vi "Update Channels.vi"(6 "Settings":T1={"Step Values"=[], "Only Execute When Test Running"=TRUE, "Reset Sequence When Test Starts"=TRUE, "Current Sequence ID"=0, "Total Iterations"=0, "Current Step Start Timestamp"=0.0, "Number of Sequence Steps"=0, "Num of Analog Channels"=0, "Num of Digital Channels"=0, "Delay Before Starting Sequence"=0.0, "Show UI"=FALSE, "Time Remaining"=0.0, "Test Running"=FALSE, "Pause Timestamp"=0.0, "Default Analog Values"=[], "Default Digital Values"=[]}, 8 "error in":errorcluster, 9 "Analog":bool, 10 "Previous Number of Channels":i32=8, 11 "Plugin in":refnum<class "Sequencer with Output Values.lvclass">) -> (0 "error out":errorcluster, 1 "Channels to Remove":string[](array[string]), 2 "Updated Number of Channels":i32, 3 "Plugin out":refnum<class "Sequencer with Output Values.lvclass">, 5 "Channels to Add":refnum<class "Producer Channel.lvclass">[](array[class]))   [LabVIEW 2020, in "Sequencer with Output Values.lvlib" / "Sequencer with Output Values.lvclass"]
uses:
  Sequencer with Output Values.lvclass
  Params.ctl
  Step Settings.ctl
  <vilib>/FlexLogger/SDK/PluginSDK.lvlibp/PEFClasses/SDK/Producer Channel/Producer Channel.lvclass
  <vilib>/FlexLogger/SDK/PluginSDK.lvlibp/PEFClasses/SDK/Channel/Data Type.ctl
  Global Strings.vi
  <vilib>/FlexLogger/SDK/PluginSDK.lvlibp/PEFClasses/SDK/Producer Channel/Create Producer Channel.vi
  <vilib>/FlexLogger/SDK/PluginSDK.lvlibp/PEFClasses/SDK/Plugin/Plugin.lvclass
  <vilib>/FlexLogger/SDK/PluginSDK.lvlibp
  <vilib>/FlexLogger/SDK/PluginSDK.lvlibp/PEFClasses/SDK/Channel/Channel.lvclass
  C:/Program Files/National Instruments/LabVIEW 2024/vi.lib/FlexLogger/SDK/PluginSDK.lvlibp/PEFClasses/SDK/Plugin/Plugin.lvclass
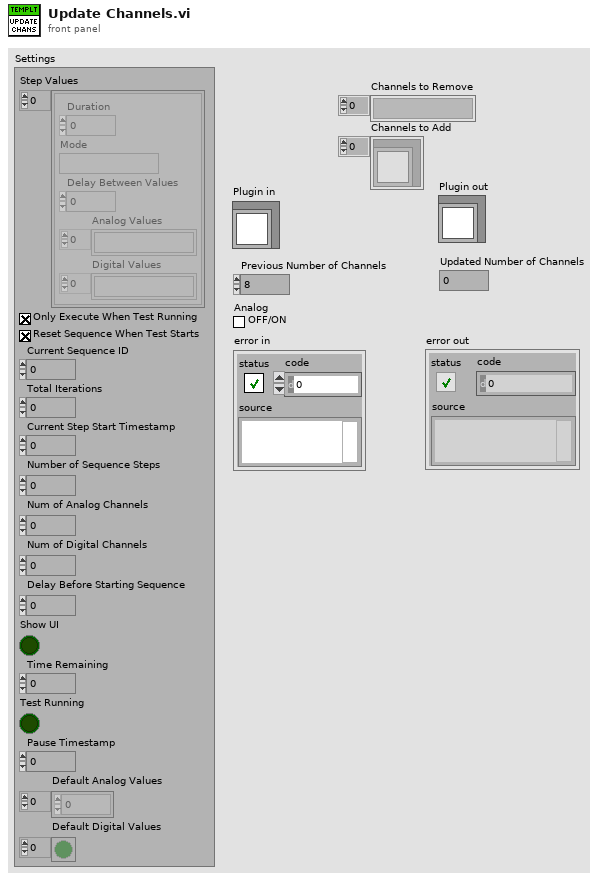
[diagram p1: front panel]
types:
  T1 = typedef "Sequencer with Output Values.lvlib/Sequencer with Output Values.lvclass/Params.ctl" = cluster{"Step Values":T2[], "Only Execute When Test Running":bool, "Reset Sequence When Test Starts":bool, "Current Sequence ID":u32, "Total Iterations":u32, "Current Step Start Timestamp":dbl, "Number of Sequence Steps":i32, "Num of Analog Channels":i32, "Num of Digital Channels":i32, "Delay Before Starting Sequence":dbl, "Show UI":bool, "Time Remaining":dbl, "Test Running":bool, "Pause Timestamp":dbl, "Default Analog Values":dbl[], "Default Digital Values":bool[]}
  T2 = typedef "Sequencer with Output Values.lvlib/Sequencer with Output Values.lvclass/Step Settings.ctl" = cluster{"Duration":dbl, "Mode":string, "Delay Between Values":dbl, "Analog Values":string[], "Digital Values":string[]}
  T3 = typedef "PluginSDK.lvlibp/Channel.lvclass/Data Type.ctl" = enum16{"Wfm (DBL)", "Wfm (Digital)"}
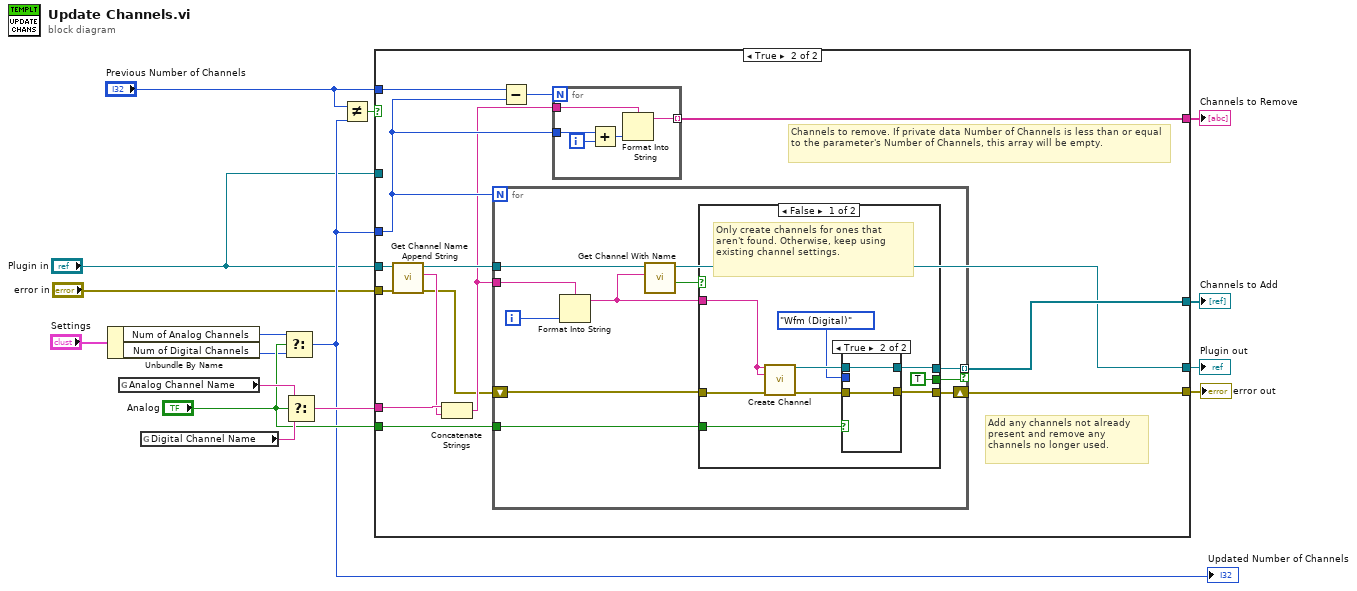
[diagram p0: block diagram]
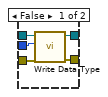
[diagram p3: hidden frame]
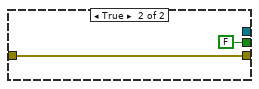
[diagram p4: hidden frame]
diagram:
  n1 = Unbundle By Name("Settings") -> ("Num of Analog Channels"=w4:i32, "Num of Digital Channels"=w3:i32)
  n2 = global read "Global Strings.vi" "Analog Channel Name"() -> (w14:string)
  n3 = global read "Global Strings.vi" "Digital Channel Name"() -> (w13:string)
  n4 = Select(t=w4, s="Analog", f=w3) -> (s? t:f=w8:i32)
  "Updated Number of Channels" <- w8
  n5 = Select(t=w14, s="Analog", f=w13) -> (s? t:f=w12:string)
  n6 = Not Equal?(x="Previous Number of Channels", y=w8) -> (x != y?=w16:bool)
  n7 = case shown="True" w16 {
    tunnel: "Previous Number of Channels" -> [_ w32]
    tunnel: w8 -> [_ w29]
    tunnel: "Plugin in" -> [w18 w25]
    tunnel: "error in" -> [w17 w21]
    tunnel: "Plugin in" -> [_ _]
    tunnel: [w18 w24] -> w11
    tunnel: [w17 w27] -> w10
    tunnel: w12 -> [_ w23]
    tunnel: "Analog" -> [_ w30]
    tunnel: [_ w28] -> w2
    tunnel: [_ w26] -> w1
    frame False {
    }
    frame True {
      # "Add any channels not already present and remove any channels no longer used."
      # "Channels to remove. If private data Number of Channels is less than or equal to the parameter's Number of Channels, this array will be empty."
      n8 = call "Get Channel Name Append String.vi"("error in (no error)"=w21, "Plugin In"=w25) -> ("error out"=w19:errorcluster, "Channel Append String"=w20:string, "Plugin Out"=w24:refnum<class "Sequencer with Output Values.lvclass">)  [unwired: 7 in]
      n9 = Concatenate Strings(w23, w20) -> (w22:string)
      n10 = for {
        N: w29 -> [_]
        tunnel: w24 -> [w42]
        tunnel: [w41] -> w26 mode=indexing if=w35
        shift-right: [w40] -> w27
        shift-left: w19 -> [w39]
        tunnel: w22 -> [w38]
        tunnel: w30 -> [w36]
        i -> [w37]
        n11 = Format Into String(format string=w38, w37) -> (resulting string=w34:string)  [unwired: 2 in, 1 out]
        n12 = call <vilib>:"Get Channel With Name.vi"("Name"=w34, "Plugin in"=w42) -> ("Found?"=w33:bool)  [unwired: 7 in, 2 out]
        n13 = case shown="False" w33 {
          tunnel: w34 -> [w49 _]
          tunnel: [w44 _] -> w41
          tunnel: [TRUE FALSE] -> w35
          tunnel: [w43 w60] -> w40
          tunnel: w39 -> [w50 w60]
          tunnel: w36 -> [w48 _]
          frame False {
            # "Only create channels for ones that aren't found. Otherwise, keep using existing channel settings."
            n14 = call-poly <vilib>:"Create Channel.vi"("Unique Channel Identifier"=w49, "Default Channel Name"=w49, "error in (no error)"=w50) -> ("Producer Channel"=w47:refnum<class "Producer Channel.lvclass">, "error out"=w45:errorcluster)  [unwired: 11 in]
            n15 = case shown="True" w48 {
              tunnel: w47 -> [w56 w58]
              tunnel: Data_Type."Wfm (Digital)" ("Data Type") -> [w55 _]
              tunnel: w45 -> [w54 w57]
              tunnel: [w53 w58] -> w44
              tunnel: [w52 w57] -> w43
              frame False {
                n16 = call-dynamic "Write Data Type.vi"("error in (no error)"=w54, "Data Type"=w55, "Channel in"=w56) -> ("error out"=w52:errorcluster, "Channel out"=w53:refnum<class "Producer Channel.lvclass">)  [unwired: 7 in]
              }
              frame True {
              }
            }
          }
          frame True {
          }
        }
      }
      n17 = Subtract(x=w32, y=w29) -> (x-y=w31:i32)
      n18 = for {
        N: w31 -> [_]
        tunnel: [w61] -> w28 mode=indexing
        tunnel: w29 -> [w64]
        tunnel: w22 -> [w62]
        i -> [w65]
        n19 = Add(x=w64, y=w65) -> (x+y=w63:i32)
        n20 = Format Into String(format string=w62, w63) -> (resulting string=w61:string)  [unwired: 2 in, 1 out]
      }
    }
  }
  "Plugin out" <- w11
  "error out" <- w10
  "Channels to Remove" <- w2
  "Channels to Add" <- w1
